vi "倒计时器.vi"() -> ()   [LabVIEW 2017]
panel:
  out "倒计时":string
  out "布尔":bool
  in  "停止":bool
  in  "开始倒计时":bool
  in  "定时时间选择":enum16{"20秒", "10秒", "6秒"}(ring)
  # "倒 计 时 器"
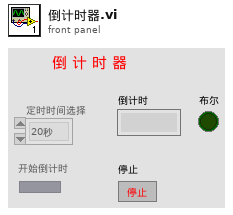
[diagram p1: front panel]
types:
  T1 = enum8{"Enabled", "Disabled", "Disabled and Grayed Out"}
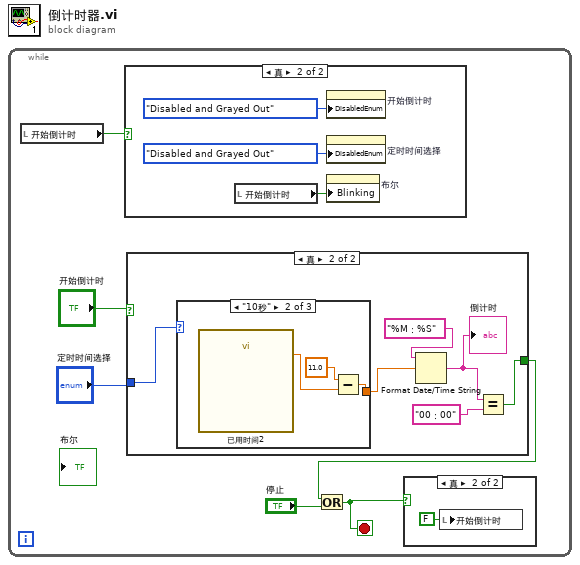
[diagram p0: block diagram]
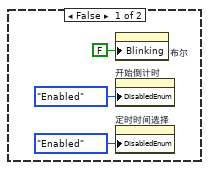
[diagram p3: hidden frame]
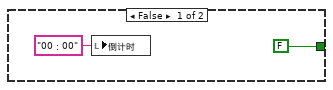
[diagram p4: hidden frame]
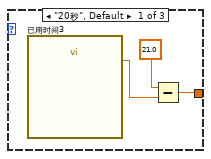
[diagram p5: hidden frame]
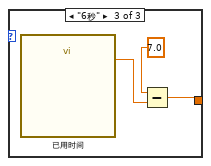
[diagram p6: hidden frame]
diagram:
  n1 = while {
    stop <- w1 stop-if-true
    n2 = local read "开始倒计时"() -> (w2:bool)
    n3 = case shown="真" w2 {
      frame False {
        n4 = property on="布尔" class="Bool (严格)"("Blinking"=FALSE ("闪烁")) -> ()  [unwired: 2 in, 2 out]
        n5 = property on="开始倒计时" class="Bool (严格)"("DisabledEnum"=T1."Enabled" ("禁用")) -> ()  [unwired: 2 in, 2 out]
        n6 = property on="定时时间选择" class="Enum (严格)"("DisabledEnum"=T1."Enabled" ("禁用")) -> ()  [unwired: 2 in, 2 out]
      }
      frame True {
        n7 = local read "开始倒计时"() -> (w13:bool)
        n8 = property on="开始倒计时" class="Bool (严格)"("DisabledEnum"=T1."Disabled and Grayed Out" ("禁用")) -> ()  [unwired: 2 in, 2 out]
        n9 = property on="定时时间选择" class="Enum (严格)"("DisabledEnum"=T1."Disabled and Grayed Out" ("禁用")) -> ()  [unwired: 2 in, 2 out]
        n10 = property on="布尔" class="Bool (严格)"("Blinking"=w13) -> ()  [unwired: 2 in, 2 out]
      }
    }
    n11 = case shown="真" "开始倒计时" {
      tunnel: [FALSE w17] -> w5
      tunnel: "定时时间选择" -> [_ w16]
      frame False {
        n12 = local write "倒计时"("00：00" ("倒计时")) -> ()
      }
      frame True {
        n13 = case shown="\"10秒\"" w16 {
          tunnel: [w22 w25 w29] -> w20
          frame "20秒", Default {
            n14 = call "已用时间3"() -> ("Elapsed Time (s)"=w24:dbl)  [unwired: 12 in, 7 out]
            n15 = Subtract(x=21.0, y=w24) -> (x-y=w22:dbl)
          }
          frame "10秒" {
            n16 = call "已用时间2"() -> ("Elapsed Time (s)"=w27:dbl)  [unwired: 12 in, 7 out]
            n17 = Subtract(x=11.0, y=w27) -> (x-y=w25:dbl)
          }
          frame "6秒" {
            n18 = call "已用时间"() -> ("Elapsed Time (s)"=w28:dbl)  [unwired: 12 in, 7 out]
            n19 = Subtract(x=7.0, y=w28) -> (x-y=w29:dbl)
          }
        }
        n20 = Format Date/Time String(time format string (%c)="%M：%S" ("时间格式字符串(%c)"), seconds (now)=w20) -> (date/time string=w19:string)  [unwired: 1 in]
        "倒计时" <- w19
        n21 = Equal?(x=w19, y="00：00") -> (x = y?=w17:bool)
      }
    }
    n22 = Or(x=w5, y="停止") -> (x .or. y?=w1:bool)
    n23 = case shown="真" w1 {
      frame False {
      }
      frame True {
        n24 = local write "开始倒计时"(FALSE) -> ()
      }
    }
  }
